vi "Open All Relays.vi"(8 "error in":errorcluster, 11 "Physical Channels":string[](array[string])=["Dev1/port0", "Dev1/port1", "Dev1/port2"]) -> (0 "error out":errorcluster)   [LabVIEW 2013]
uses:
  <vilib>/DAQmx/create/channels.llb/DAQmx Create Channel (DO-Digital Output).vi
  <vilib>/DAQmx/write.llb/DAQmx Write (Digital 1D U32 NChan 1Samp).vi
  <resource>/objmgr/daqmx.rc
panel:
  in  "initial value":u32
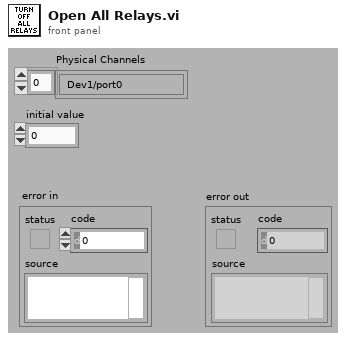
[diagram p1: front panel]
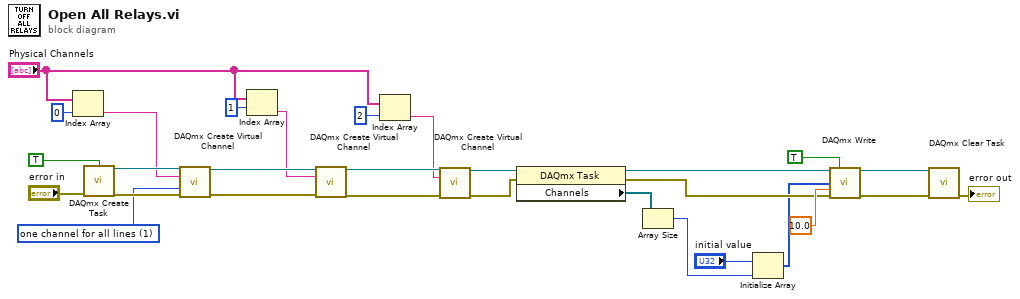
[diagram p0: block diagram]
diagram:
  w20 = 1 items=["one channel for each line", "one channel for all lines"] ("line grouping")
  n1 = Index Array(array="Physical Channels", index=0) -> (element=w14:string)
  n2 = call <vilib>:"DAQmx Create Task.vi"("auto cleanup"=TRUE, "error in"="error in") -> ("task out"=w26:refnum<k21>, "error out"=w27:errorcluster)  [unwired: 12 in]
  n3 = call-poly <vilib>:"DAQmx Create Virtual Channel.vi"("task in"=w26, "lines"=w14, "line grouping"=w20, "error in"=w27) -> ("task out"=w18:refnum<k21>, "error out"=w19:errorcluster)  [unwired: 10 in]
  n4 = Index Array(array="Physical Channels", index=1) -> (element=w12:string)
  n5 = call-poly <vilib>:"DAQmx Create Virtual Channel.vi"("task in"=w18, "lines"=w12, "error in"=w19) -> ("task out"=w16:refnum<k21>, "error out"=w17:errorcluster)  [unwired: 11 in]
  n6 = Index Array(array="Physical Channels", index=2) -> (element=w10:string)
  n7 = call-poly <vilib>:"DAQmx Create Virtual Channel.vi"("task in"=w16, "lines"=w10, "error in"=w17) -> ("task out"=w6:refnum<k21>, "error out"=w5:errorcluster)  [unwired: 11 in]
  n8 = property class="DAQmx Task"(reference=w6, error in=w5) -> (reference out=w3:refnum<k21>, error out=w2:errorcluster, "Channels"=w4:refnum<k21>[])
  n9 = Array Size(array=w4) -> (size(s)=w8:i32)
  n10 = Initialize Array("initial value", w8) -> (w1:u32[])
  n11 = call-poly <vilib>:"DAQmx Write.vi"("task/channels in"=w3, "auto start"=TRUE, "data"=w1, "timeout"=10.0, "error in"=w2) -> ("task out"=w22:refnum<k21>, "error out"=w23:errorcluster)  [unwired: 8 in, 1 out]
  n12 = call <vilib>:"DAQmx Clear Task.vi"("task in"=w22, "error in"=w23) -> ("error out"=→"error out":errorcluster)  [unwired: 13 in]
